vi "ModStarted.vi"(10 "StartArgs":T1, 11 "FGVWithEventTrace":refnum<class "FGVWithEventTrace.lvclass">) -> ()   [LabVIEW 2024, in "FGVWithEventTrace.lvclass"]
uses:
  FGVWithEventTrace.lvclass
  DebugTraceHandle/StartArgs.ctl
  Command.ctl
  DebugTraceHandle/DebugTraceHandle.lvclass
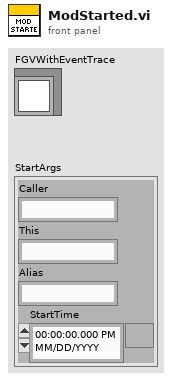
[diagram p1: front panel]
types:
  T1 = typedef "DebugTraceHandle.lvclass/StartArgs.ctl" = cluster{"Caller":string, "This":string, "Alias":string, "StartTime":timestamp}
  T2 = typedef "FGVWithEventTrace.lvclass/Command.ctl" = enum16{"Add", "Get", "Remove", "Clear"}
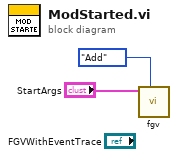
[diagram p0: block diagram]
diagram:
  n1 = call "fgv.vi"("Command"=Command."Add", "StartArgs"="StartArgs") -> ()  [unwired: 8 in, 2 out]
